vi "Compare VIs.vi"() -> ()   [LabVIEW 2026, in "VILab.lvlib"]
uses:
  VILab.lvlib
  CTLs/Resource.ctl
panel:
  out "Array 3":string[](array[string])
  out "Array 2":string[](array[string])
  out "Array":i32[](array[numeric])
  out "System":T1[](array[typedef])
  out "Modern":T1[](array[typedef])
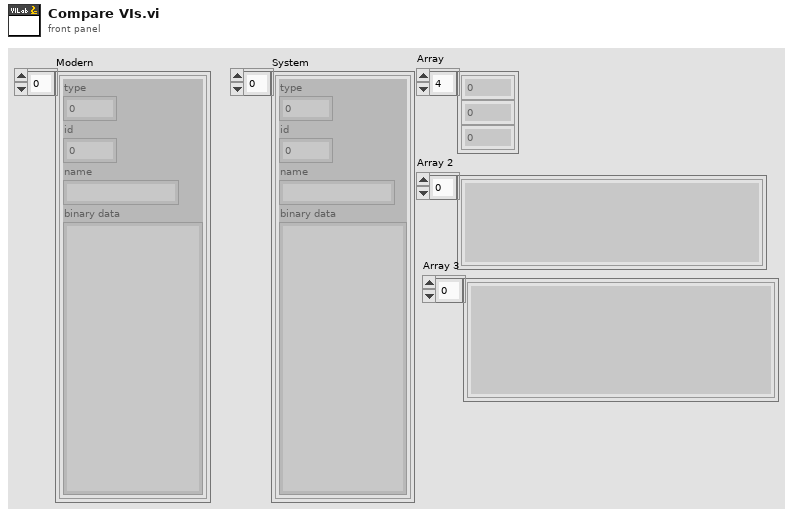
[diagram p1: front panel]
types:
  T1 = typedef "VILab.lvlib/Resource.ctl" = cluster{"type":u32, "id":i32, "name":string, "binary data":string}
  T2 = cluster{"type":bool, "id":bool, "name":bool, "binary data":bool}
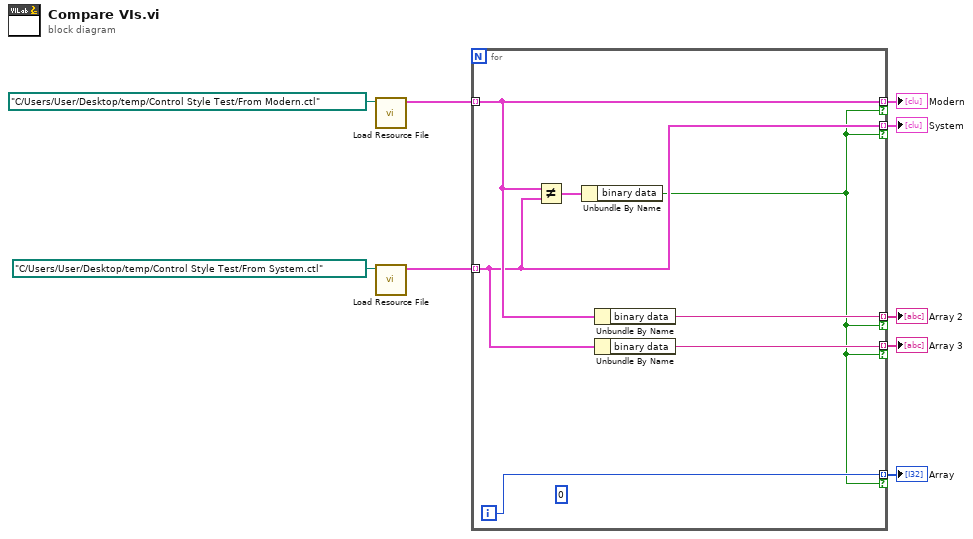
[diagram p0: block diagram]
diagram:
  n1 = call "Load Resource File.vi"("Resource File"=path "C:/Users/User/Desktop/temp/Control Style Test/From Modern.ctl") -> ("Resources"=w7:T1[])  [unwired: 8 in, 2 out]
  n2 = call "Load Resource File.vi"("Resource File"=path "C:/Users/User/Desktop/temp/Control Style Test/From System.ctl") -> ("Resources"=w6:T1[])  [unwired: 8 in, 2 out]
  n3 = for {
    tunnel: w7 -> [w14] mode=indexing
    tunnel: w6 -> [w13] mode=indexing
    tunnel: [w14] -> w5 mode=indexing if=w10
    tunnel: [w13] -> w4 mode=indexing if=w10
    tunnel: [w15] -> w3 mode=indexing if=w10
    tunnel: [w12] -> w2 mode=indexing if=w10
    tunnel: [w11] -> w1 mode=indexing if=w10
    i -> [w15]
    (unwired) 0
    n4 = Not Equal?(x=w14, y=w13) -> (x != y?=w16:T2)
    n5 = Unbundle By Name(w16) -> ("binary data"=w10:bool)
    n6 = Unbundle By Name(w14) -> ("binary data"=w12:string)
    n7 = Unbundle By Name(w13) -> ("binary data"=w11:string)
  }
  "Modern" <- w5
  "System" <- w4
  "Array" <- w3
  "Array 2" <- w2
  "Array 3" <- w1
